vi "manualoverride_deel2 (SubVI).vi"(10 "snelheidsverdeling":dbl(slide) scale=-5.0..5.0, 11 "snelheid":dbl(slide) scale=0.0..10.0) -> (1 "rechtermotor na":dbl, 2 "linkermotor na":dbl)   [LabVIEW 2019]
uses:
  <vilib>/myRIO/Express VI/Onboard IO/PWM/PWM Express VI.xnode
  <vilib>/myRIO/Instrument Drivers/Onboard IO/PWM/vis/Set Duty Cycle and Frequency.vi
  <vilib>/myRIO/Instrument Drivers/Onboard IO/PWM/PWM.lvlib
  <vilib>/myRIO/Instrument Drivers/Onboard IO/PWM/typedefs/PWM Configuration.ctl
  <vilib>/myRIO/Common/Instrument Driver Framework/myRIO v1.0/PWM/typedefs/PWM Channels Enum.ctl
  <vilib>/myRIO/Common/Instrument Driver Framework/Utilities/typedefs/Generic FPGA Reference.ctl
  <vilib>/myRIO/Common/Instrument Driver Framework/Utilities/typedefs/myRIO v1.0 Reference.ctl
  <vilib>/myRIO/Common/Instrument Driver Framework/Utilities/typedefs/Hardware Version Enum.ctl
  <vilib>/myRIO/Common/Instrument Driver Framework/Utilities/typedefs/myRIO Generic Hardware Reference.ctl
  <vilib>/myRIO/Instrument Drivers/Onboard IO/PWM/typedefs/PWM Reference.ctl
  <vilib>/myRIO/Instrument Drivers/Onboard IO/PWM/vis/myRIO PWM Open.xnode
  <vilib>/myRIO/Common/Instrument Driver Framework/Utilities/vis/Is FPGA Ref Available.vi
  <vilib>/myRIO/Common/Instrument Driver Framework/myRIO v1.0/PWM/vis/myRIO v1.1 Open PWM.vi
  <vilib>/userDefined/High Color/nirio_resource_hc.ctl
panel:
  out "Numeric":dbl
  # "naar rechts"
  # "naar links"
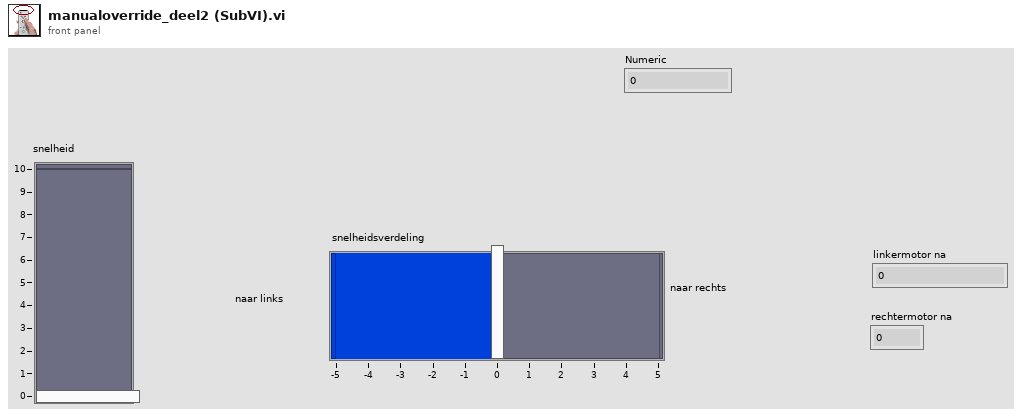
[diagram p1: front panel]
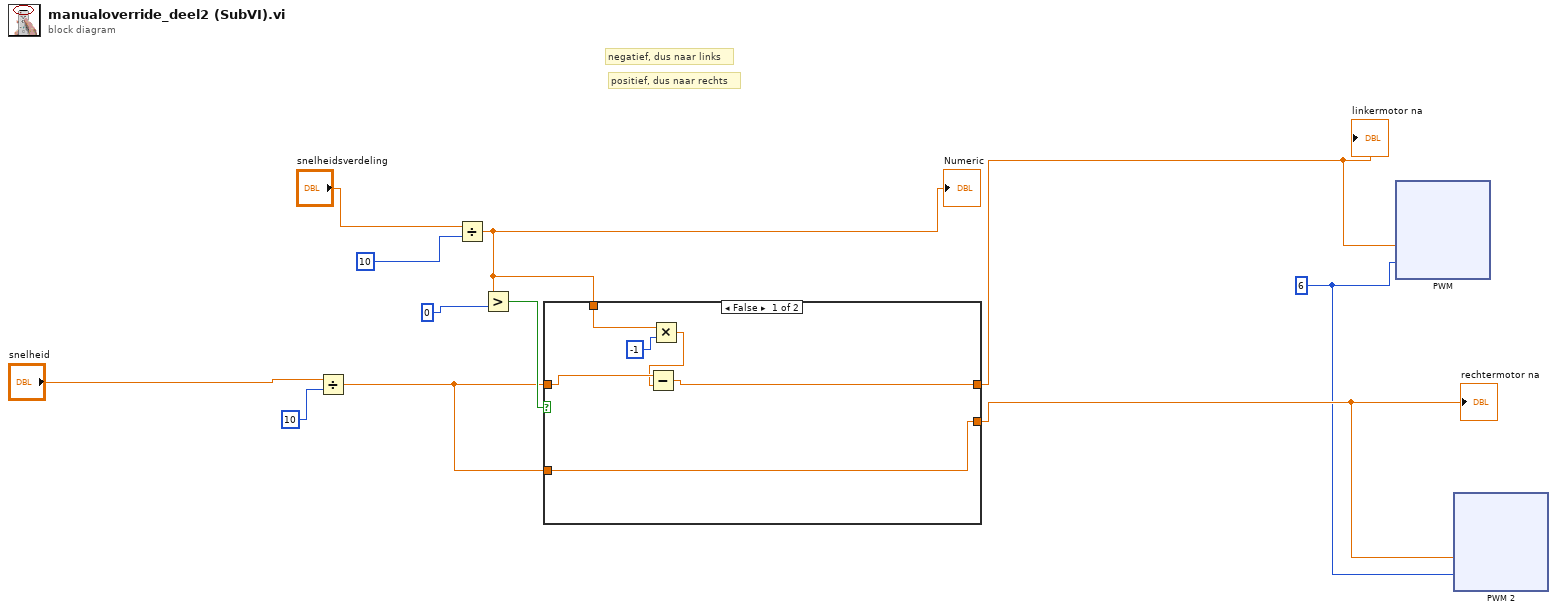
[diagram p0: block diagram]
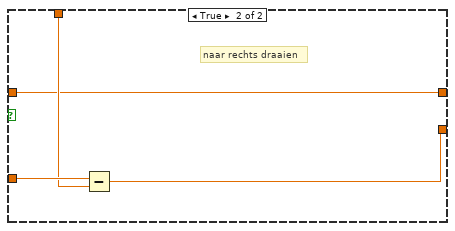
[diagram p2: hidden frame]
diagram:
  w1 = 6
  # "positief, dus naar rechts"
  # "negatief, dus naar links"
  n1 = Divide(x="snelheid", y=10) -> (x/y=w5:dbl)
  n2 = Divide(x="snelheidsverdeling", y=10) -> (x/y=w4:dbl)
  "Numeric" <- w4
  n3 = Greater?(x=w4, y=0) -> (0:w7:bool)
  n4 = case shown="False" w7 {
    tunnel: w5 -> [w17 w18]
    tunnel: w5 -> [w15 w21]
    tunnel: [w15 w19] -> w3
    tunnel: w4 -> [w14 w20]
    tunnel: [w16 w18] -> w2
    frame False {
      n5 = Multiply(x=w14, y=-1) -> (x*y=w12:dbl)
      n6 = Subtract(x=w17, y=w12) -> (x-y=w16:dbl)
    }
    frame True {
      # "naar rechts draaien"
      n7 = Subtract(x=w21, y=w20) -> (x-y=w19:dbl)
    }
  }
  "rechtermotor na" <- w3
  "linkermotor na" <- w2
  n8 = xnode "PWM"("Duty Cycle"=w2, "Frequency [Hz]"=w1) -> ()  [unwired: 1 in, 1 out]
  n9 = xnode "PWM 2"("Duty Cycle"=w3, "Frequency [Hz]"=w1) -> ()  [unwired: 1 in, 1 out]
